vi "TREE_Get First Child Only Tag.vi"(8 "error in":errorcluster, 10 "Parent Tag":string, 11 "Tree Ref":refnum<vi>) -> (0 "error out":errorcluster, 2 "tag out":string)   [LabVIEW 2016]
doc: "Set a customize symbol for a item. Notice that all the symbol of items have the same symbol index will change. Set a new symbol index if you want to customize a single item."
panel:
  # "Input"
  # "Output"
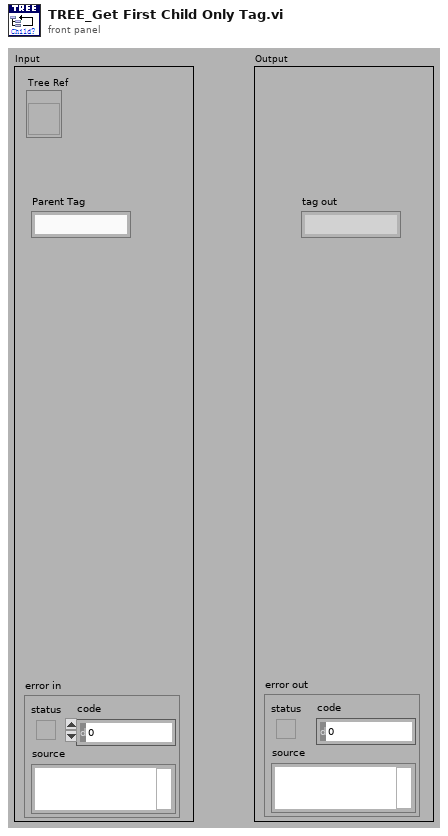
[diagram p1: front panel]
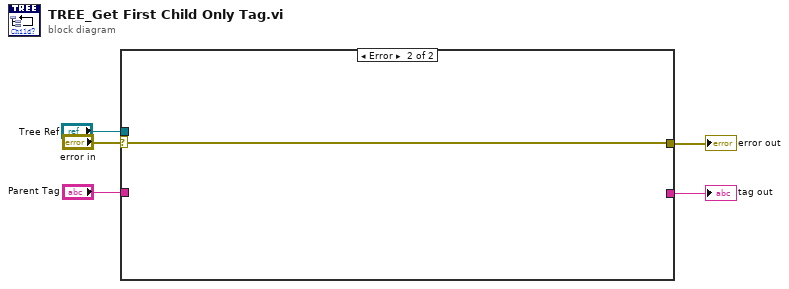
[diagram p0: block diagram]
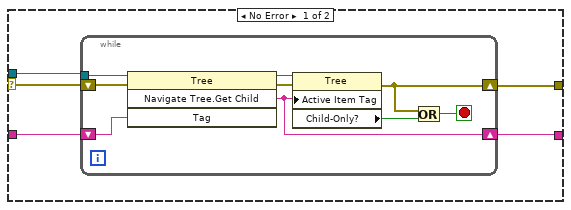
[diagram p2: hidden frame]
diagram:
  n1 = case shown="Error" "error in" {
    selector: "error in" -> [w10 w20]
    tunnel: [w6 w20] -> w5
    tunnel: "Tree Ref" -> [w9 _]
    tunnel: "Parent Tag" -> [w8 _]
    tunnel: [w7 _] -> w1
    frame No Error {
      n2 = while {
        tunnel: w9 -> [w19]
        shift-right: [w13] -> w7
        shift-left: w8 -> [w17]
        shift-right: [w11] -> w6
        shift-left: w10 -> [w18]
        stop <- w12 stop-if-true
        n3 = invoke class="Tree" method="Navigate Tree.Get Child"(reference=w19, error in=w18, "Tag"=w17) -> (reference out=w16:refnum<vi>, error out=w15:errorcluster, "Navigate Tree:Get Child"=w13:string)  [unwired: 1 in, 1 out]
        n4 = property class="Tree"(reference=w16, error in=w15, "Active Item Tag"=w13) -> (error out=w11:errorcluster, "Child-Only?"=w14:bool)  [unwired: 1 out]
        n5 = Or(x=w11, y=w14) -> (x .or. y?=w12:bool)
      }
    }
    frame Error {
    }
  }
  "error out" <- w5
  "tag out" <- w1
